vi "Initalize (seq）(SubVI).vi"(10 "字符串":string, 11 "簇":T1={"initialize"=enum."SR830", "6221"={"6221 Resource"="GPIB0::24::INSTR", "Delta status"=FALSE, "电流|RMS(A)"=0.0}, "SR830+6221"={"source"=0, "Current(A)"=0.0, "阻抗(Ohm)"=0.0, "SR830 1"=FALSE, "SR830 2"=FALSE, "SR830 3"=FALSE, "SR830 4"=FALSE, "VISA 1"="", "VISA 2"="", "VISA 3"="", "VISA 4"="", "Reserve 1"=0, "Reserve 2"=-1, "Reserve 3"=-1, "Reserve 4"=-1, "Sensitivity 1"=-1, "Sensitivity 2"=0, "Sensitivity 3"=-1, "Sensitivity 4"=-1, "量程入 1"=0, "量程入 2"=0, "量程入 3"=0, "量程入 4"=0}, "2400"={"2400"=FALSE, "VISA"="GPIB0::9::INSTR", "Output Level (0)"=1e-05, "Compliance  Level (0.1)"=10.0}, "ch"={"ch"=[], "current"=[], "change?"=[], "holding current\nwhen change ch?"=FALSE}, "Instrument"={"335 Resource"="GPIB0::24::INSTR", "Input (0:A)"=0, "Instrument Type"=enum."SVSM", "quantum design"=refnum, "Heater Output (1:1)"=1, "semaphore"=refnum, "TCP master instance"=refnum, "335 Status"=refnum, "M24C Resource"="GPIB0::24::INSTR", "4G supply"="GPIB0::24::INSTR", "Temp Status 24C"=refnum, "Temp"=refnum, "9T信号"=refnum, "limit"={"Field limit"=0.0, "Field rate limit"=0.0, "Temp limit"=0.0, "Temp low limit"=0.0, "Temp rate limit "=0.0}, "4g supply status"=refnum, "vi路径"=""}, "Aborting"=refnum, "数据文件"=refnum, "warning"=refnum, "2614B"={"2614B chA"=FALSE, "2614B chB"=FALSE, "VISA"=""}, "33522b"={"33522b resource name"="GPIB0::16::INSTR", "零电压"=0.0, "最大电压"=148.0, "间隔"=4.0, "最小电压"=-48.0, "PZT Scan?"=FALSE}} {"Instrument"."Input (0:A)" items=["A", "B"]; "Instrument"."Heater Output (1:1)" items=["1"=1, "2"=2]; "SR830+6221"."Sensitivity 4" items=["Auto Gain"=-1, "2 nV/fA"=0, "5 nV/fA"=1, "10 nV/fA"=2, "20 nV/fA"=3, "50 nV/fA"=4, "100 nV/fA"=5, "200 nV/fA"=6, "500 nV/fA"=7, "1 uV/pA"=8, "2 uV/pA"=9, "5 uV/pA"=10, "10 uV/pA"=11, "20 uV/pA"=12, "50 uV/pA"=13, "100 uV/pA"=14, "200 uV/pA"=15, "500 uV/pA"=16, "1 mV/nA"=17, "2 mV/nA"=18, "5 mV/nA"=19, "10 mV/nA"=20, "20 mV/nA"=21, "50 mV/nA"=22, "100 mV/nA"=23, "200 mV/nA"=24, "500 mV/mA"=25, "1 V/uA"=26]; "SR830+6221"."Sensitivity 3" items=["Auto Gain"=-1, "2 nV/fA"=0, "5 nV/fA"=1, "10 nV/fA"=2, "20 nV/fA"=3, "50 nV/fA"=4, "100 nV/fA"=5, "200 nV/fA"=6, "500 nV/fA"=7, "1 uV/pA"=8, "2 uV/pA"=9, "5 uV/pA"=10, "10 uV/pA"=11, "20 uV/pA"=12, "50 uV/pA"=13, "100 uV/pA"=14, "200 uV/pA"=15, "500 uV/pA"=16, "1 mV/nA"=17, "2 mV/nA"=18, "5 mV/nA"=19, "10 mV/nA"=20, "20 mV/nA"=21, "50 mV/nA"=22, "100 mV/nA"=23, "200 mV/nA"=24, "500 mV/mA"=25, "1 V/uA"=26]; "SR830+6221"."Sensitivity 1" items=["Auto Gain"=-1, "2 nV/fA"=0, "5 nV/fA"=1, "10 nV/fA"=2, "20 nV/fA"=3, "50 nV/fA"=4, "100 nV/fA"=5, "200 nV/fA"=6, "500 nV/fA"=7, "1 uV/pA"=8, "2 uV/pA"=9, "5 uV/pA"=10, "10 uV/pA"=11, "20 uV/pA"=12, "50 uV/pA"=13, "100 uV/pA"=14, "200 uV/pA"=15, "500 uV/pA"=16, "1 mV/nA"=17, "2 mV/nA"=18, "5 mV/nA"=19, "10 mV/nA"=20, "20 mV/nA"=21, "50 mV/nA"=22, "100 mV/nA"=23, "200 mV/nA"=24, "500 mV/mA"=25, "1 V/uA"=26]; "SR830+6221"."Sensitivity 2" items=["Auto Gain"=-1, "2 nV/fA"=0, "5 nV/fA"=1, "10 nV/fA"=2, "20 nV/fA"=3, "50 nV/fA"=4, "100 nV/fA"=5, "200 nV/fA"=6, "500 nV/fA"=7, "1 uV/pA"=8, "2 uV/pA"=9, "5 uV/pA"=10, "10 uV/pA"=11, "20 uV/pA"=12, "50 uV/pA"=13, "100 uV/pA"=14, "200 uV/pA"=15, "500 uV/pA"=16, "1 mV/nA"=17, "2 mV/nA"=18, "5 mV/nA"=19, "10 mV/nA"=20, "20 mV/nA"=21, "50 mV/nA"=22, "100 mV/nA"=23, "200 mV/nA"=24, "500 mV/mA"=25, "1 V/uA"=26]; "SR830+6221"."Reserve 4" items=["Auto Gain"=-1, "2 nV/fA"=0, "5 nV/fA"=1, "10 nV/fA"=2, "20 nV/fA"=3, "50 nV/fA"=4, "100 nV/fA"=5, "200 nV/fA"=6, "500 nV/fA"=7, "1 uV/pA"=8, "2 uV/pA"=9, "5 uV/pA"=10, "10 uV/pA"=11, "20 uV/pA"=12, "50 uV/pA"=13, "100 uV/pA"=14, "200 uV/pA"=15, "500 uV/pA"=16, "1 mV/nA"=17, "2 mV/nA"=18, "5 mV/nA"=19, "10 mV/nA"=20, "20 mV/nA"=21, "50 mV/nA"=22, "100 mV/nA"=23, "200 mV/nA"=24, "500 mV/mA"=25, "1 V/uA"=26]; "SR830+6221"."Reserve 3" items=["Auto Reserve"=-1, "High Reserve"=0, "Normal"=1, "Low Noise"=2]; "SR830+6221"."Reserve 2" items=["Auto Reserve"=-1, "High Reserve"=0, "Normal"=1, "Low Noise"=2]; "SR830+6221"."Reserve 1" items=["Auto Reserve"=-1, "High Reserve"=0, "Normal"=1, "Low Noise"=2]; "SR830+6221"."source" items=["SR830 1", "SR830 2", "SR830 3", "SR830 4"]}) -> (3 "输出簇":T1={"initialize"=enum."SR830", "6221"={"6221 Resource"="GPIB0::24::INSTR", "Delta status"=FALSE, "电流|RMS(A)"=0.0}, "SR830+6221"={"source"=0, "Current(A)"=0.0, "阻抗(Ohm)"=0.0, "SR830 1"=FALSE, "SR830 2"=FALSE, "SR830 3"=FALSE, "SR830 4"=FALSE, "VISA 1"="", "VISA 2"="", "VISA 3"="", "VISA 4"="", "Reserve 1"=0, "Reserve 2"=-1, "Reserve 3"=-1, "Reserve 4"=-1, "Sensitivity 1"=-1, "Sensitivity 2"=0, "Sensitivity 3"=-1, "Sensitivity 4"=-1, "量程入 1"=0, "量程入 2"=0, "量程入 3"=0, "量程入 4"=0}, "2400"={"2400"=FALSE, "VISA"="", "Output Level (0)"=1e-05, "Compliance  Level (0.1)"=10.0}, "ch"={"ch"=[], "current"=[], "change?"=[], "holding current\nwhen change ch?"=FALSE}, "Instrument"={"335 Resource"="GPIB0::24::INSTR", "Input (0:A)"=0, "Instrument Type"=enum."SVSM", "quantum design"=refnum, "Heater Output (1:1)"=1, "semaphore"=refnum, "TCP master instance"=refnum, "335 Status"=refnum, "M24C Resource"="GPIB0::24::INSTR", "4G supply"="GPIB0::24::INSTR", "Temp Status 24C"=refnum, "Temp"=refnum, "9T信号"=refnum, "limit"={"Field limit"=0.0, "Field rate limit"=0.0, "Temp limit"=0.0, "Temp low limit"=0.0, "Temp rate limit "=0.0}, "4g supply status"=refnum, "vi路径"=""}, "Aborting"=refnum, "数据文件"=refnum, "warning"=refnum, "2614B"={"2614B chA"=FALSE, "2614B chB"=FALSE, "VISA"=""}, "33522b"={"33522b resource name"="", "零电压"=0.0, "最大电压"=148.0, "间隔"=4.0, "最小电压"=-48.0, "PZT Scan?"=FALSE}} {"Instrument"."Input (0:A)" items=["A", "B"]; "Instrument"."Heater Output (1:1)" items=["1"=1, "2"=2]; "SR830+6221"."Sensitivity 4" items=["Auto Gain"=-1, "2 nV/fA"=0, "5 nV/fA"=1, "10 nV/fA"=2, "20 nV/fA"=3, "50 nV/fA"=4, "100 nV/fA"=5, "200 nV/fA"=6, "500 nV/fA"=7, "1 uV/pA"=8, "2 uV/pA"=9, "5 uV/pA"=10, "10 uV/pA"=11, "20 uV/pA"=12, "50 uV/pA"=13, "100 uV/pA"=14, "200 uV/pA"=15, "500 uV/pA"=16, "1 mV/nA"=17, "2 mV/nA"=18, "5 mV/nA"=19, "10 mV/nA"=20, "20 mV/nA"=21, "50 mV/nA"=22, "100 mV/nA"=23, "200 mV/nA"=24, "500 mV/mA"=25, "1 V/uA"=26]; "SR830+6221"."Sensitivity 3" items=["Auto Gain"=-1, "2 nV/fA"=0, "5 nV/fA"=1, "10 nV/fA"=2, "20 nV/fA"=3, "50 nV/fA"=4, "100 nV/fA"=5, "200 nV/fA"=6, "500 nV/fA"=7, "1 uV/pA"=8, "2 uV/pA"=9, "5 uV/pA"=10, "10 uV/pA"=11, "20 uV/pA"=12, "50 uV/pA"=13, "100 uV/pA"=14, "200 uV/pA"=15, "500 uV/pA"=16, "1 mV/nA"=17, "2 mV/nA"=18, "5 mV/nA"=19, "10 mV/nA"=20, "20 mV/nA"=21, "50 mV/nA"=22, "100 mV/nA"=23, "200 mV/nA"=24, "500 mV/mA"=25, "1 V/uA"=26]; "SR830+6221"."Sensitivity 1" items=["Auto Gain"=-1, "2 nV/fA"=0, "5 nV/fA"=1, "10 nV/fA"=2, "20 nV/fA"=3, "50 nV/fA"=4, "100 nV/fA"=5, "200 nV/fA"=6, "500 nV/fA"=7, "1 uV/pA"=8, "2 uV/pA"=9, "5 uV/pA"=10, "10 uV/pA"=11, "20 uV/pA"=12, "50 uV/pA"=13, "100 uV/pA"=14, "200 uV/pA"=15, "500 uV/pA"=16, "1 mV/nA"=17, "2 mV/nA"=18, "5 mV/nA"=19, "10 mV/nA"=20, "20 mV/nA"=21, "50 mV/nA"=22, "100 mV/nA"=23, "200 mV/nA"=24, "500 mV/mA"=25, "1 V/uA"=26]; "SR830+6221"."Sensitivity 2" items=["Auto Gain"=-1, "2 nV/fA"=0, "5 nV/fA"=1, "10 nV/fA"=2, "20 nV/fA"=3, "50 nV/fA"=4, "100 nV/fA"=5, "200 nV/fA"=6, "500 nV/fA"=7, "1 uV/pA"=8, "2 uV/pA"=9, "5 uV/pA"=10, "10 uV/pA"=11, "20 uV/pA"=12, "50 uV/pA"=13, "100 uV/pA"=14, "200 uV/pA"=15, "500 uV/pA"=16, "1 mV/nA"=17, "2 mV/nA"=18, "5 mV/nA"=19, "10 mV/nA"=20, "20 mV/nA"=21, "50 mV/nA"=22, "100 mV/nA"=23, "200 mV/nA"=24, "500 mV/mA"=25, "1 V/uA"=26]; "SR830+6221"."Reserve 4" items=["Auto Gain"=-1, "2 nV/fA"=0, "5 nV/fA"=1, "10 nV/fA"=2, "20 nV/fA"=3, "50 nV/fA"=4, "100 nV/fA"=5, "200 nV/fA"=6, "500 nV/fA"=7, "1 uV/pA"=8, "2 uV/pA"=9, "5 uV/pA"=10, "10 uV/pA"=11, "20 uV/pA"=12, "50 uV/pA"=13, "100 uV/pA"=14, "200 uV/pA"=15, "500 uV/pA"=16, "1 mV/nA"=17, "2 mV/nA"=18, "5 mV/nA"=19, "10 mV/nA"=20, "20 mV/nA"=21, "50 mV/nA"=22, "100 mV/nA"=23, "200 mV/nA"=24, "500 mV/mA"=25, "1 V/uA"=26]; "SR830+6221"."Reserve 3" items=["Auto Reserve"=-1, "High Reserve"=0, "Normal"=1, "Low Noise"=2]; "SR830+6221"."Reserve 2" items=["Auto Reserve"=-1, "High Reserve"=0, "Normal"=1, "Low Noise"=2]; "SR830+6221"."Reserve 1" items=["Auto Reserve"=-1, "High Reserve"=0, "Normal"=1, "Low Noise"=2]; "SR830+6221"."source" items=["SR830 1", "SR830 2", "SR830 3", "SR830 4"]})   [LabVIEW 2019, in "Take Seq.lvlib"]
uses:
  Take Seq.lvlib
  ctl/config.ctl
  <vilib>/NI/Modbus Library/API/Master/Modbus Master.lvclass
  ctl/initialize.ctl
  ctl/Instrument.ctl
  ctl/Instrument Type.ctl
  C:/Users/Admin/Desktop/measure/lib/QDInstrument.dll
  lib/QDInstrument.dll
  ctl/335 state.ctl
  ctl/limit.ctl
  ctl/9T mag field stauts.ctl
  ctl/warning.ctl
  initialize.lvlib
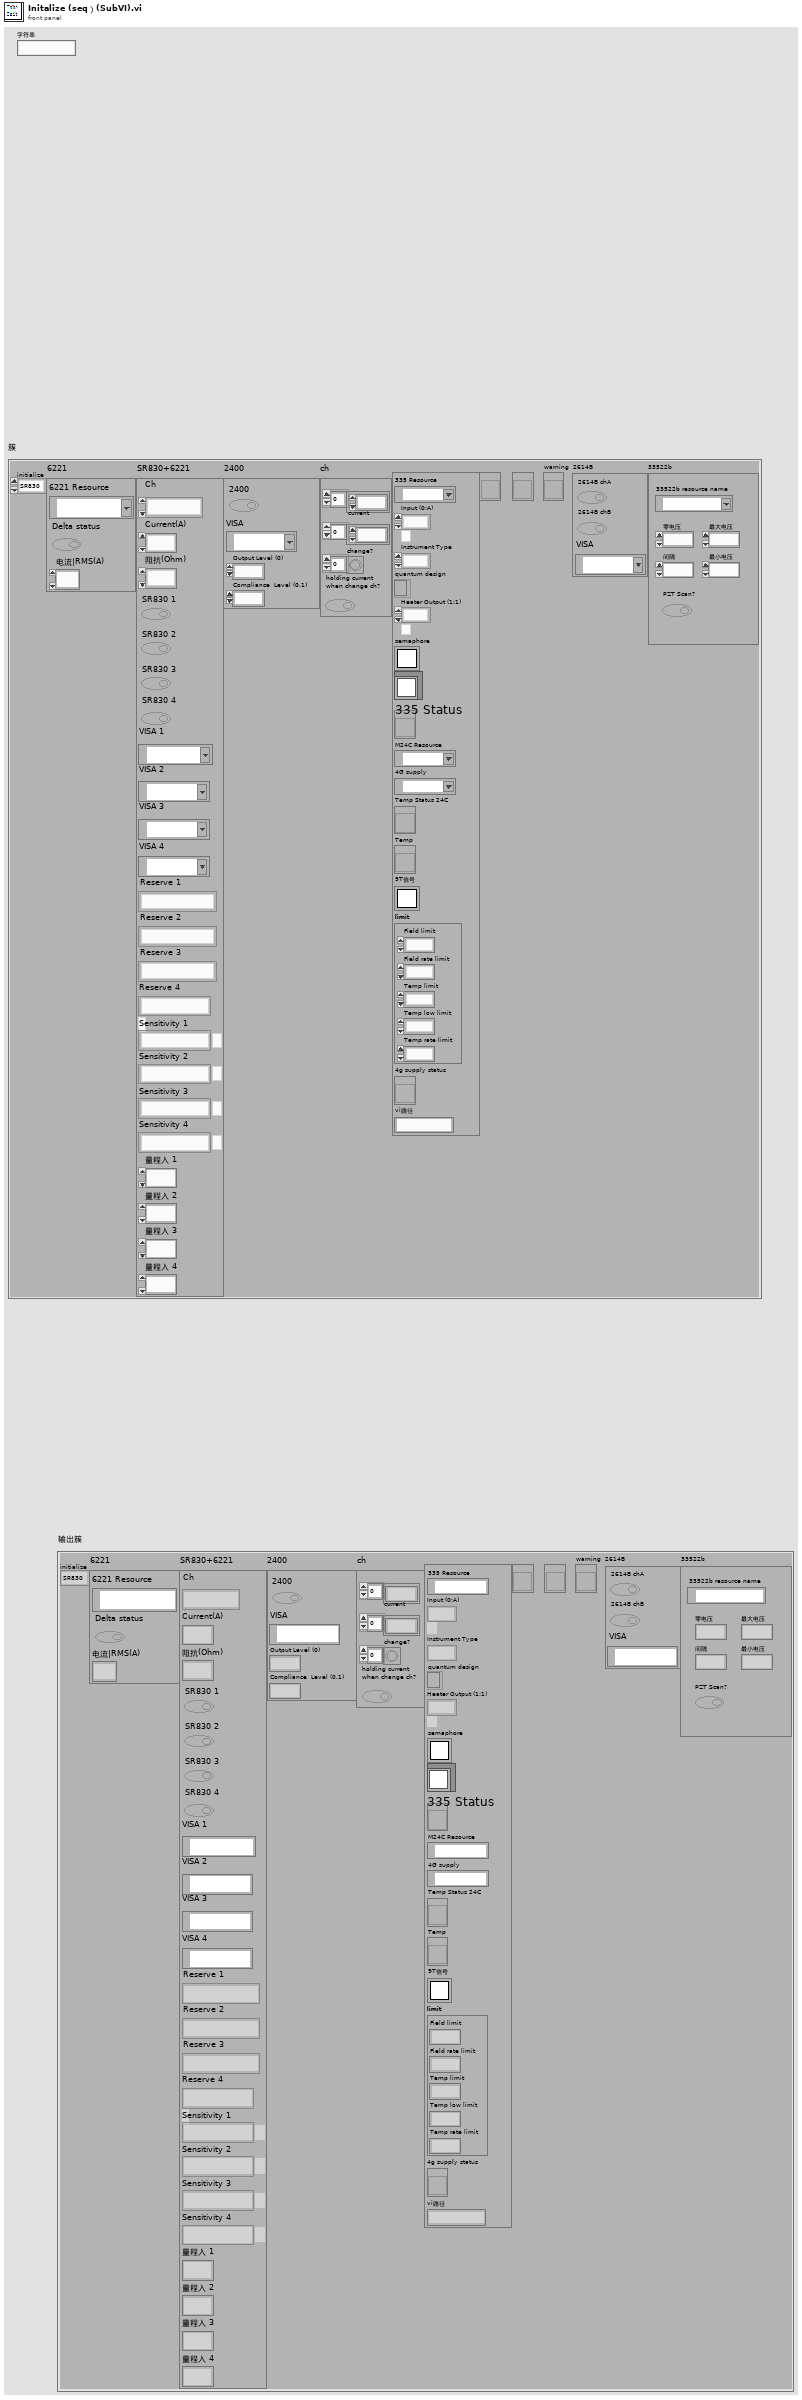
[diagram p1: front panel]
types:
  T1 = typedef "config.ctl" = cluster{"initialize":T2, "6221":cluster{"6221 Resource":refnum<visa-resource-name>, "Delta status":bool, "电流|RMS(A)":dbl}, "SR830+6221":cluster{"source":u16, "Current(A)":dbl, "阻抗(Ohm)":dbl, "SR830 1":bool, "SR830 2":bool, "SR830 3":bool, "SR830 4":bool, "VISA 1":refnum<visa-resource-name>, "VISA 2":refnum<visa-resource-name>, "VISA 3":refnum<visa-resource-name>, "VISA 4":refnum<visa-resource-name>, "Reserve 1":i16, "Reserve 2":i16, "Reserve 3":i16, "Reserve 4":i16, "Sensitivity 1":i16, "Sensitivity 2":i16, "Sensitivity 3":i16, "Sensitivity 4":i16, "量程入 1":i32, "量程入 2":i32, "量程入 3":i32, "量程入 4":i32}, "2400":cluster{"2400":bool, "VISA":refnum<visa-resource-name>, "Output Level (0)":dbl, "Compliance  Level (0.1)":dbl}, "ch":cluster{"ch":i32[], "current":dbl[], "change?":bool[], "holding current\nwhen change ch?":bool}, "Instrument":T3, "Aborting":refnum<vi>, "数据文件":refnum<vi>, "warning":refnum<vi>, "2614B":cluster{"2614B chA":bool, "2614B chB":bool, "VISA":refnum<visa-resource-name>}, "33522b":cluster{"33522b resource name":refnum<visa-resource-name>, "零电压":dbl, "最大电压":dbl, "间隔":dbl, "最小电压":dbl, "PZT Scan?":bool}}
  T2 = typedef "initialize.ctl" = enum16{"SR830", "keithley6221-SR830", "Delta", "Delta-tunnelling", "keithley6221-2182-DC", "PZT"}
  T3 = typedef "Instrument.ctl" = cluster{"335 Resource":refnum<visa-resource-name>, "Input (0:A)":u16, "Instrument Type":T4, "quantum design":refnum<k24>, "Heater Output (1:1)":u16, "semaphore":T5, "TCP master instance":refnum<class "Modbus Master.lvclass">, "335 Status":refnum<vi>, "M24C Resource":refnum<visa-resource-name>, "4G supply":refnum<visa-resource-name>, "Temp Status 24C":refnum<vi>, "Temp":refnum<vi>, "9T信号":T5, "limit":T6, "4g supply status":refnum<vi>, "vi路径":string}
  T4 = typedef "Instrument Type.ctl" = enum16{"PPMS", "VersaLab", "DynaCool", "SVSM", "PPMS-Rotate", "Lakeshore335", "9T mag"}
  T5 = typedef "Semaphore RefNum" = refnum<k1>
  T6 = typedef "limit.ctl" = cluster{"Field limit":dbl, "Field rate limit":dbl, "Temp limit":dbl, "Temp low limit":dbl, "Temp rate limit ":dbl}
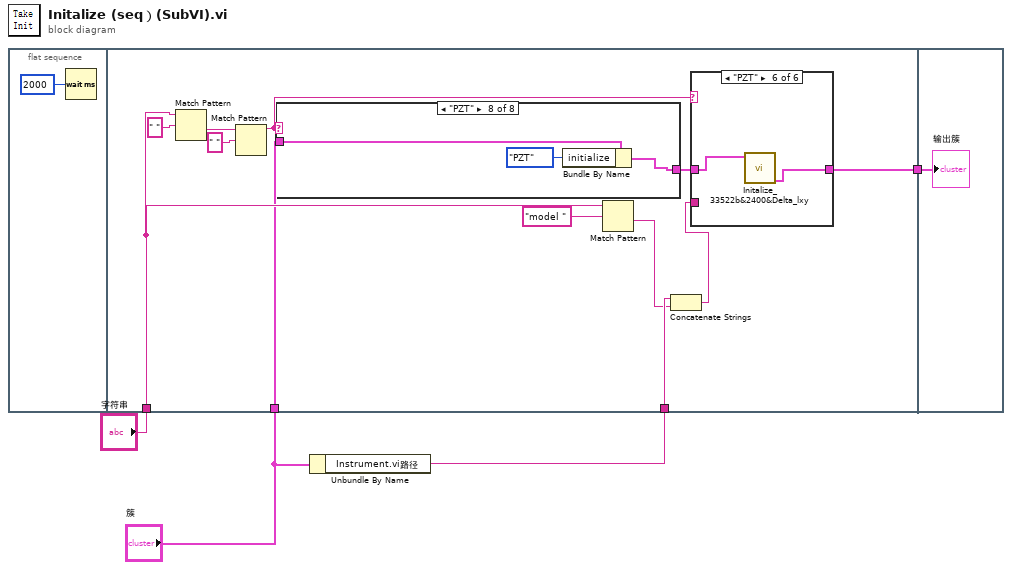
[diagram p0: block diagram]
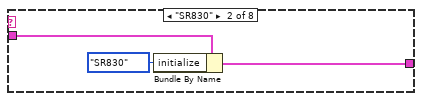
[diagram p3: hidden frame]
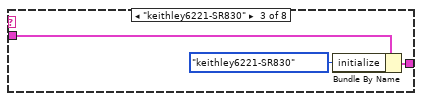
[diagram p4: hidden frame]
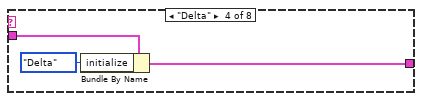
[diagram p5: hidden frame]
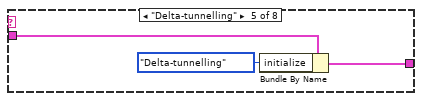
[diagram p6: hidden frame]
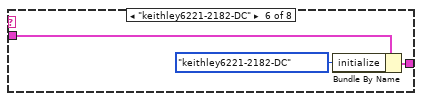
[diagram p7: hidden frame]
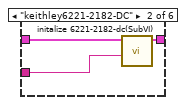
[diagram p10: hidden frame]
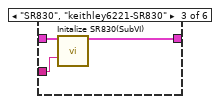
[diagram p11: hidden frame]
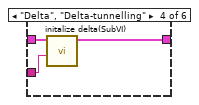
[diagram p12: hidden frame]
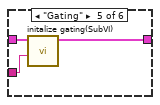
[diagram p13: hidden frame]
diagram:
  n1 = flat-sequence {
    tunnel: "字符串" -> [w15]
    tunnel: "簇" -> [w11]
    tunnel: [w13] -> w3
    tunnel: w1 -> [w7]
    tunnel: w3 -> [w53]
    frame #0 {
      n2 = Wait (ms)(milliseconds to wait=u32 2000) -> ()  [unwired: 1 out]
    }
    frame #1 {
      n3 = Match Pattern(string=w15, regular expression=" " ("正则表达式")) -> (after substring=w16:string)  [unwired: 1 in, 3 out]
      n4 = Match Pattern(string=w16, regular expression=" " ("正则表达式")) -> (before substring=w12:string)  [unwired: 1 in, 3 out]
      n5 = case shown="\"PZT\"" w12 {
        tunnel: w11 -> [w18 w21 w24 w27 w29 w32 w34 w37]
        tunnel: [w18 w20 w23 w26 w30 w33 w34 w36] -> w10
        frame "假", Default {
        }
        frame "SR830" {
          n6 = Bundle By Name(cluster=w21, "initialize"=initialize."SR830") -> (w20:T1)
        }
        frame "keithley6221-SR830" {
          n7 = Bundle By Name(cluster=w24, "initialize"=initialize."keithley6221-SR830") -> (w23:T1)
        }
        frame "Delta" {
          n8 = Bundle By Name(cluster=w27, "initialize"=initialize."Delta") -> (w26:T1)
        }
        frame "Delta-tunnelling" {
          n9 = Bundle By Name(cluster=w29, "initialize"=initialize."Delta-tunnelling") -> (w30:T1)
        }
        frame "keithley6221-2182-DC" {
          n10 = Bundle By Name(cluster=w32, "initialize"=initialize."keithley6221-2182-DC") -> (w33:T1)
        }
        frame "Gating" {
        }
        frame "PZT" {
          n11 = Bundle By Name(cluster=w37, "initialize"=initialize."PZT") -> (w36:T1)
        }
      }
      n12 = Match Pattern(string=w15, regular expression="model " ("正则表达式")) -> (after substring=w6:string)  [unwired: 1 in, 3 out]
      n13 = Concatenate Strings(w7, w6) -> (w8:string)
      n14 = case shown="\"PZT\"" w12 {
        tunnel: w8 -> [_ w39 w44 w47 w50 _]
        tunnel: w10 -> [w38 w41 w43 w46 w49 w52]
        tunnel: [w38 w40 w42 w45 w48 w51] -> w13
        frame "假", Default {
        }
        frame "keithley6221-2182-DC" {
          n15 = call "initalize 6221-2182-dc(SubVI).vi"("字符串"=w39, "簇"=w41) -> ("输出簇"=w40:T1)  [unwired: 9 in]
        }
        frame "SR830", "keithley6221-SR830" {
          n16 = call "Initalize SR830(SubVI).vi"("簇"=w43, "字符串"=w44) -> ("输出簇"=w42:T1)  [unwired: 13 in]
        }
        frame "Delta", "Delta-tunnelling" {
          n17 = call "initalize delta(SubVI).vi"("字符串"=w47, "簇"=w46) -> ("输出簇"=w45:T1)  [unwired: 9 in]
        }
        frame "Gating" {
          n18 = call "initalize gating(SubVI).vi"("簇"=w49, "字符串"=w50) -> ("输出簇"=w48:T1)  [unwired: 8 in]
        }
        frame "PZT" {
          n19 = call "Initalize_33522b&2400&Delta_lxy.vi"("config"=w52) -> ("输出簇"=w51:T1)  [unwired: 10 in]
        }
      }
    }
    frame #2 {
      "输出簇" <- w53
    }
  }
  n20 = Unbundle By Name("簇") -> ("Instrument.vi路径"=w1:string)
